vi "Bits to Bytes1.vi"(11 "bits":bool[](array[boolean])) -> (2 "count":u8, 3 "bytes":u8[](array[numeric]))   [LabVIEW 2021, in "NI_modbus_upd.lvlib"]
uses:
  NI_modbus_upd.lvlib
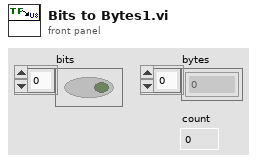
[diagram p1: front panel]
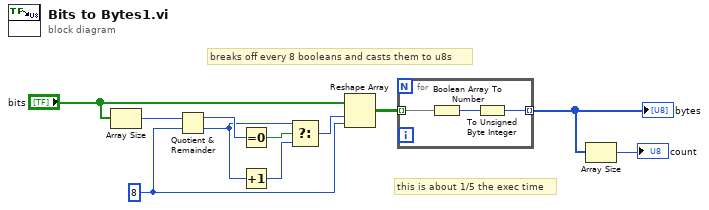
[diagram p0: block diagram]
diagram:
  w2 = 8 ("y")
  # "this is about 1/5 the exec time"
  # "breaks off every 8 booleans and casts them to u8s"
  n1 = Array Size(array="bits") -> (size(s)=w8:i32)
  n2 = Quotient & Remainder(x=w8, y=w2) -> (x-y*floor(x/y)=w7:i32, floor(x/y)=w4:i32)
  n3 = Equal To 0?(x=w7) -> (x = 0?=w6:bool)
  n4 = Increment(x=w4) -> (x+1=w5:i32)
  n5 = Select(t=w4, s=w6, f=w5) -> (s? t:f=w3:i32)
  n6 = Reshape Array("bits", w3, w2) -> (w1:bool[][])
  n7 = for {
    tunnel: w1 -> [w13] mode=indexing
    tunnel: [w14] -> w10 mode=indexing
    n8 = Boolean Array To Number(Boolean array=w13) -> (number=w12:u32)
    n9 = To Unsigned Byte Integer(number=w12) -> (unsigned 8bit integer=w14:u8)
  }
  "bytes" <- w10
  n10 = Array Size(array=w10) -> (size(s)=→"count":i32)
